vi "Cam_project_ROI.vi"() -> ()   [LabVIEW 2018]
uses:
  <vilib>/userdefined/High Color/IMAQdx.ctl
  <vilib>/vision/driver/NI_Vision_Acquisition_Software.lvlib
panel:
  out "Frame Rate 2":dbl
  out "error out":errorcluster
  out "Acquired Frames/s":dbl
  out "Distance of the object":dbl
  out "Frame Rate":dbl(knob) scale=0.0..10.0
  out "Case":cluster{i32, i32}(graph)
  out "Detection":cluster{i16, i16}(graph)
  out "cluster":T1
  out "Array":i32[](array[numeric])
  out "Numeric":i32
  out "Area of the Bounding Rectangle":i32
  out "?":T2(plugin-control)
  out "Binary Image":T2(plugin-control)
  out "?":bool
  in  "?":dbl(slide)=100.0 scale=0.0..1000.0
  out "?":T3(array[cluster]) {"Score" format="%.2f"; "Centroid"."y" format="%.2f"; "Centroid"."x" format="%.2f"}
  out "Detected:":i32
  in  "Stop":bool
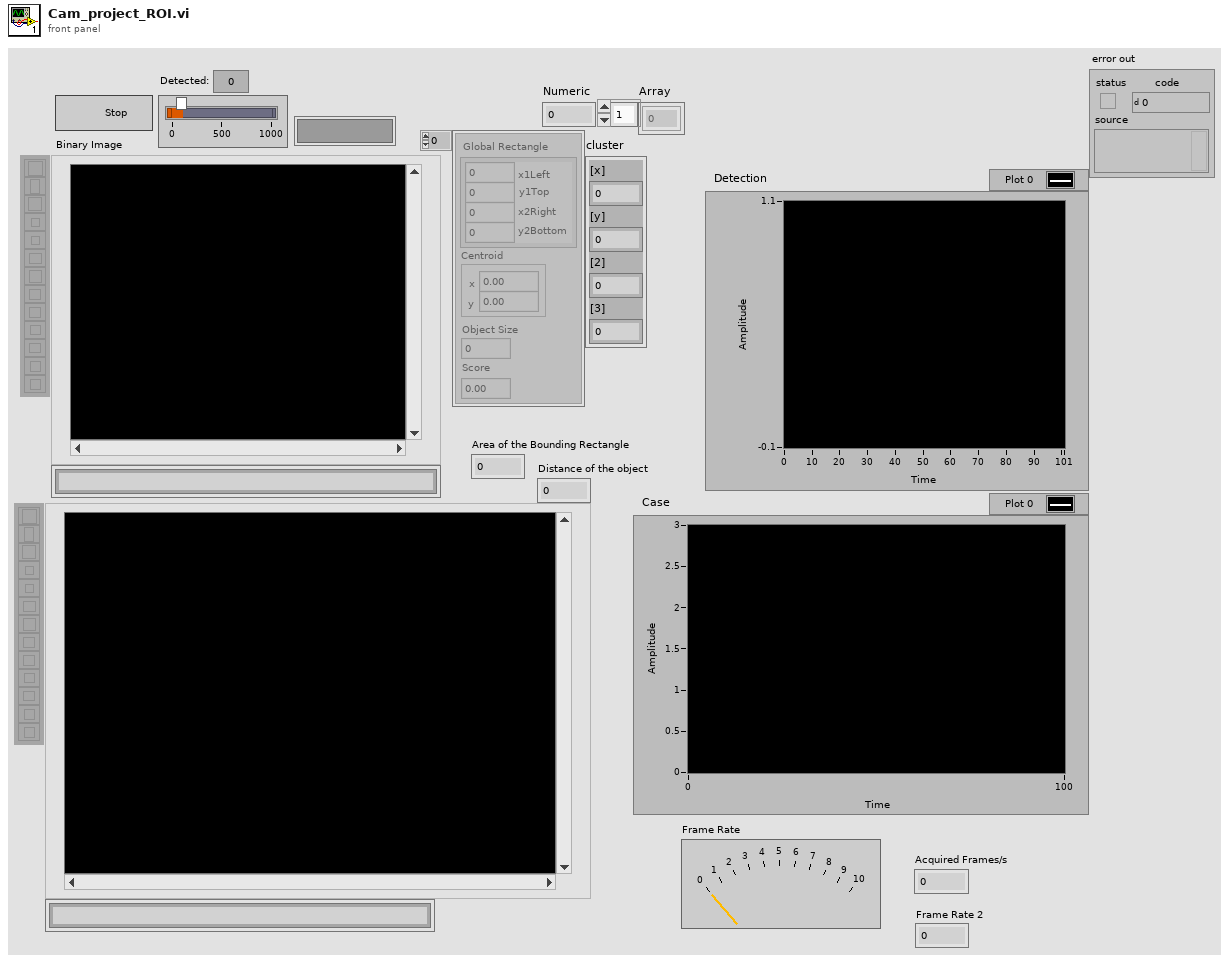
[diagram p1: front panel]
types:
  T1 = cluster{"[x]":sgl, "[y]":sgl, "[2]":sgl, "[3]":sgl}
  T2 = typedef "IMAQ Image.ctl" = refnum<image>
  T3 = cluster{"Global Rectangle":cluster{"x1Left":i32, "y1Top":i32, "x2Right":i32, "y2Bottom":i32}, "Centroid":cluster{"x":sgl, "y":sgl}, "Object Size":u32, "Score":dbl}[]
  T4 = typedef "IMAQdx.ctl" = refnum<k21>
  T5 = cluster{"Desired Font (Application)":enum16{"User-specified Font", "Application Font", "System Font", "Dialog Font"}, "[User-specified Font]":cluster{"Font Name":string, "Size":i16, "Strikeout?":bool, "Italic?":bool, "Underline?":bool, "Outline?":bool, "Shadow?":bool, "Bold?":bool, "Rotation Angle":dbl}, "Horizontal Alignment":i16, "Vertical Alignment":i16}
  T6 = enum32{"No Selection", "Point", "Line", "Rectangle", "Oval", "Polygon", "Free", "Unused1", "Unused2", "Unused3", "Broken Line", "Free Hand Line"}
  T7 = cluster{"[0]":sgl, "[1]":sgl, "[2]":sgl, "[3]":sgl}
  T8 = cluster{"[0]":dbl, "[1]":dbl, "[2]":dbl, "[3]":dbl}
  T9 = cluster{"ID":enum32{"External", "Internal"}, "Type":enum32{"No Selection", "Point", "Line", "Rectangle", "Oval", "Polygon", "Free", "Unused1", "Unused2", "Unused3", "Broken Line", "Free Hand Line"}, dbl[]}
  T10 = cluster{"ID":enum32{"External", "Internal"}, "Type":enum32{"No Selection", "Point", "Line", "Rectangle", "Oval", "Polygon", "Free", "Unused1", "Unused2", "Unused3", "Broken Line", "Free Hand Line"}, dbl[]}[]
  T11 = cluster{dbl[], cluster{"ID":enum32{"External", "Internal"}, "Type":enum32{"No Selection", "Point", "Line", "Rectangle", "Oval", "Polygon", "Free", "Unused1", "Unused2", "Unused3", "Broken Line", "Free Hand Line"}, dbl[]}[]}
  T12 = cluster{"Shape Report (Shape Detect)[0]":cluster{"Global Rectangle":cluster{"x1Left":i32, "y1Top":i32, "x2Right":i32, "y2Bottom":i32}, "Centroid":cluster{"x":sgl, "y":sgl}, "Object Size":u32, "Score":dbl}, "Shape Report (Shape Detect)[1]":cluster{"Global Rectangle":cluster{"x1Left":i32, "y1Top":i32, "x2Right":i32, "y2Bottom":i32}, "Centroid":cluster{"x":sgl, "y":sgl}, "Object Size":u32, "Score":dbl}, "Shape Report (Shape Detect)[2]":cluster{"Global Rectangle":cluster{"x1Left":i32, "y1Top":i32, "x2Right":i32, "y2Bottom":i32}, "Centroid":cluster{"x":sgl, "y":sgl}, "Object Size":u32, "Score":dbl}, "Shape Report (Shape Detect)[3]":cluster{"Global Rectangle":cluster{"x1Left":i32, "y1Top":i32, "x2Right":i32, "y2Bottom":i32}, "Centroid":cluster{"x":sgl, "y":sgl}, "Object Size":u32, "Score":dbl}, "Shape Report (Shape Detect)[4]":cluster{"Global Rectangle":cluster{"x1Left":i32, "y1Top":i32, "x2Right":i32, "y2Bottom":i32}, "Centroid":cluster{"x":sgl, "y":sgl}, "Object Size":u32, "Score":dbl}, "Shape Report (Shape Detect)[5]":cluster{"Global Rectangle":cluster{"x1Left":i32, "y1Top":i32, "x2Right":i32, "y2Bottom":i32}, "Centroid":cluster{"x":sgl, "y":sgl}, "Object Size":u32, "Score":dbl}, "Shape Report (Shape Detect)[6]":cluster{"Global Rectangle":cluster{"x1Left":i32, "y1Top":i32, "x2Right":i32, "y2Bottom":i32}, "Centroid":cluster{"x":sgl, "y":sgl}, "Object Size":u32, "Score":dbl}, "Shape Report (Shape Detect)[7]":cluster{"Global Rectangle":cluster{"x1Left":i32, "y1Top":i32, "x2Right":i32, "y2Bottom":i32}, "Centroid":cluster{"x":sgl, "y":sgl}, "Object Size":u32, "Score":dbl}, "Shape Report (Shape Detect)[8]":cluster{"Global Rectangle":cluster{"x1Left":i32, "y1Top":i32, "x2Right":i32, "y2Bottom":i32}, "Centroid":cluster{"x":sgl, "y":sgl}, "Object Size":u32, "Score":dbl}}
  T13 = cluster{"x1Left":i32, "y1Top":i32, "x2Right":i32, "y2Bottom":i32}
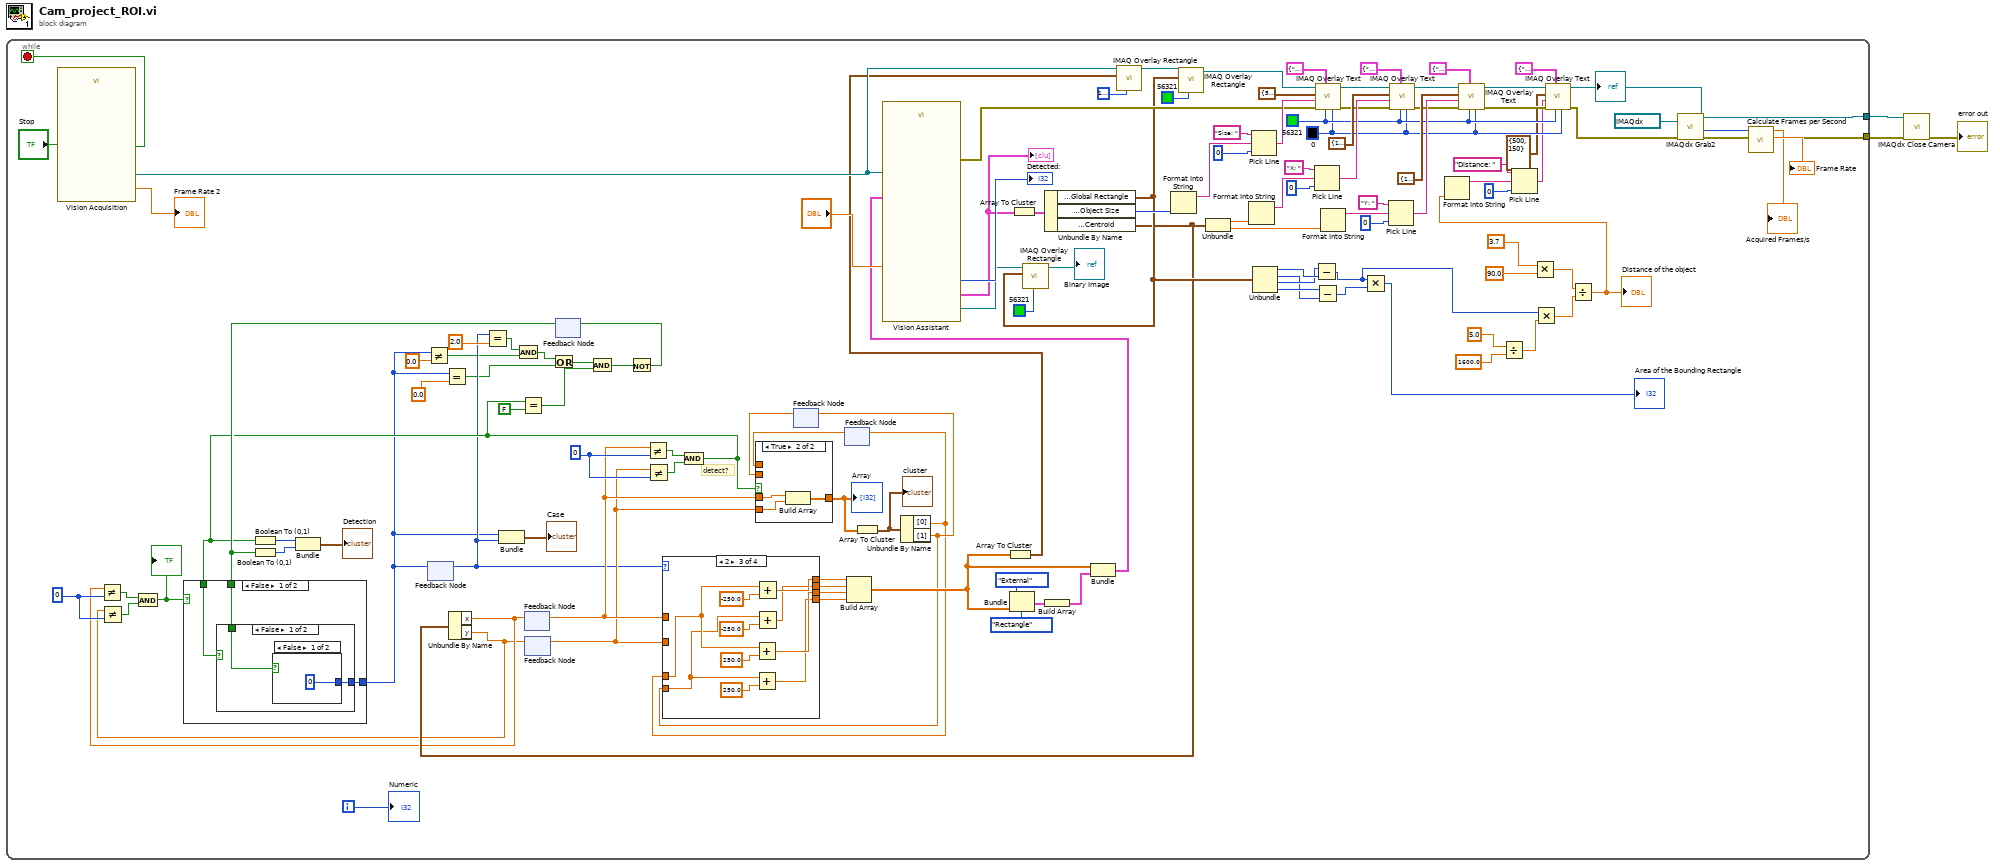
[diagram p0: block diagram]
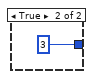
[diagram p2: hidden frame]
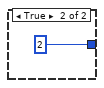
[diagram p3: hidden frame]
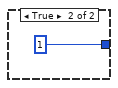
[diagram p4: hidden frame]
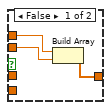
[diagram p5: hidden frame]
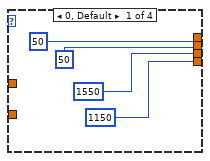
[diagram p6: hidden frame]
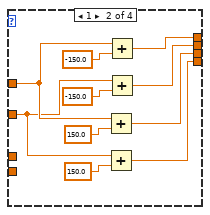
[diagram p7: hidden frame]
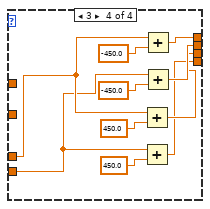
[diagram p8: hidden frame]
diagram:
  n1 = while {
    tunnel: [w8] -> w3
    tunnel: [w5] -> w2
    i -> [w56]
    stop <- w128 stop-if-true
    w66 = 0
    w71 = 0
    w17 = u32 0 ("BG Color (Transparent)")
    w18 = u32 56321 ("Text Color (black)")
    # "detect?"
    n2 = call "Vision Acquisition"("Stop (F)"="Stop") -> ("Image Out"=w81:T2, "Frame Rate"=→"Frame Rate 2":dbl, "Stopped"=w128:bool)  [unwired: 23 in, 1 out]
    n3 = feedback #1() -> (w45:i32)  [unwired: 1 in]
    n4 = Equal?(x=w45, y=sgl 2.0) -> (x = y?=w43:bool)
    n5 = feedback #2() -> (w63:sgl)  [unwired: 1 in]
    n6 = feedback #3() -> (w62:sgl)  [unwired: 1 in]
    n7 = feedback #4() -> (w52:bool)  [unwired: 1 in]
    n8 = Boolean To (0,1)(Boolean=w52) -> (0, 1=w51:i16)
    n9 = Not Equal?(x=w63, y=w66) -> (x != y?=w65:bool)
    n10 = Not Equal?(x=w62, y=w66) -> (x != y?=w64:bool)
    n11 = And(x=w65, y=w64) -> (x .and. y?=w46:bool)
    n12 = Boolean To (0,1)(Boolean=w46) -> (0, 1=w42:i16)
    n13 = Bundle(w42, w51) -> (→"Detection":cluster{i16, i16})  [unwired: 1 in]
    n14 = Equal?(x=w46, y=FALSE) -> (x = y?=w55:bool)
    n15 = feedback #5() -> (w59:sgl)  [unwired: 1 in]
    n16 = feedback #6() -> (w60:sgl)  [unwired: 1 in]
    n17 = case shown="True" w46 {
      tunnel: w63 -> [_ w143]
      tunnel: w62 -> [_ w142]
      tunnel: [w140 w141] -> w61
      tunnel: w60 -> [w138 _]
      tunnel: w59 -> [w139 _]
      frame False {
        n18 = Build Array(w138, w139) -> (w140:sgl[])
      }
      frame True {
        n19 = Build Array(w143, w142) -> (w141:sgl[])
      }
    }
    "Array" <- w61
    n20 = Array To Cluster(array=w61) -> (cluster=w33:T7)
    "cluster" <- w33
    n21 = Unbundle By Name(w33) -> ("[0]"=w57:sgl, "[1]"=w58:sgl)
    n22 = case shown="2" w45 {
      tunnel: [50 ("line index") w156 w163 w171] -> w77
      tunnel: [50 ("line index") w154 w162 w170] -> w76
      tunnel: [1550 ("line index") w150 w161 w169] -> w75
      tunnel: [1150 ("line index") w151 w160 w168] -> w74
      tunnel: w63 -> [_ w149 _ _]
      tunnel: w62 -> [_ w148 _ _]
      tunnel: w58 -> [_ _ w158 w172]
      tunnel: w57 -> [_ _ w159 w173]
      frame 0, Default {
      }
      frame 1 {
        n23 = Add(x=w149, y=150.0) -> (x+y=w150:dbl)
        n24 = Add(x=w148, y=150.0) -> (x+y=w151:dbl)
        n25 = Add(x=w149, y=-150.0) -> (x+y=w156:dbl)
        n26 = Add(x=w148, y=-150.0) -> (x+y=w154:dbl)
      }
      frame 2 {
        n27 = Add(x=w159, y=250.0) -> (x+y=w161:dbl)
        n28 = Add(x=w158, y=250.0) -> (x+y=w160:dbl)
        n29 = Add(x=w159, y=-250.0) -> (x+y=w163:dbl)
        n30 = Add(x=w158, y=-250.0) -> (x+y=w162:dbl)
      }
      frame 3 {
        n31 = Add(x=w173, y=450.0) -> (x+y=w169:dbl)
        n32 = Add(x=w172, y=450.0) -> (x+y=w168:dbl)
        n33 = Add(x=w173, y=-450.0) -> (x+y=w171:dbl)
        n34 = Add(x=w172, y=-450.0) -> (x+y=w170:dbl)
      }
    }
    n35 = feedback-in #5(w58) -> ()
    n36 = feedback-in #6(w57) -> ()
    n37 = Build Array(w77, w76, w75, w74) -> (w82:dbl[])
    n38 = Array To Cluster(array=w82) -> (cluster=w78:T8)
    n39 = Bundle("ID"=enum32{"External", "Internal"}."External", "Type"=T6."Rectangle", w82) -> (w85:T9)  [unwired: 1 in]
    n40 = Build Array(w85) -> (w84:T10)
    n41 = Bundle(w82, w84) -> (w83:T11)  [unwired: 1 in]
    n42 = call "Vision Assistant"("Image In"=w81, "Minimal Score (Shape Detect)"="?", "ROI Descriptor (Define ROI)"=w83) -> ("Image Out"=w92:T2, "Number of Matches (Shape Detect)"=→"Detected:":i32, "Shape Report (Shape Detect)"=w123:T3, "error out"=w90:errorcluster)  [unwired: 21 in]
    "?" <- w123
    n43 = Array To Cluster(array=w123) -> (cluster=w124:T12)
    n44 = Unbundle By Name(w124) -> ("Shape Report (Shape Detect)[0].Global Rectangle"=w68:T13, "Shape Report (Shape Detect)[0].Object Size"=w121:u32, "Shape Report (Shape Detect)[0].Centroid"=w67:cluster{"x":sgl, "y":sgl})
    n45 = Unbundle By Name(w67) -> ("x"=w49:sgl, "y"=w48:sgl)
    n46 = Not Equal?(x=w49, y=w71) -> (x != y?=w70:bool)
    n47 = Not Equal?(x=w48, y=w71) -> (x != y?=w69:bool)
    n48 = And(x=w70, y=w69) -> (x .and. y?=w47:bool)
    "?" <- w47
    n49 = case shown="False" w47 {
      tunnel: [w131 1] -> w39
      tunnel: w52 -> [w129 _]
      tunnel: w46 -> [w130 _]
      frame False {
        n50 = case shown="False" w130 {
          tunnel: [w133 2] -> w131
          tunnel: w129 -> [w132 _]
          frame False {
            n51 = case shown="False" w132 {
              tunnel: [0 3] -> w133
              frame False {
              }
              frame True {
              }
            }
          }
          frame True {
          }
        }
      }
      frame True {
      }
    }
    n52 = Not Equal?(x=w39, y=0.0) -> (x != y?=w38:bool)
    n53 = feedback-in #1(w39) -> ()
    n54 = Equal?(x=w39, y=0.0) -> (x = y?=w36:bool)
    n55 = Bundle(w39, w45) -> (→"Case":cluster{i32, i32})  [unwired: 1 in]
    n56 = And(x=w43, y=w38) -> (x .and. y?=w37:bool)
    n57 = feedback-in #2(w49) -> ()
    n58 = feedback-in #3(w48) -> ()
    n59 = Or(x=w37, y=w36) -> (x .or. y?=w35:bool)
    n60 = And(x=w35, y=w55) -> (x .and. y?=w41:bool)
    n61 = Not(x=w41) -> (.not. x?=w34:bool)
    n62 = feedback-in #4(w34) -> ()
    n63 = call "IMAQ Overlay Rectangle"("Color"=u32 56321, "Rectangle"=w68, "Image"=w92) -> ("Image Out"=→"Binary Image":T2)  [unwired: 7 in, 1 out]
    n64 = call "IMAQ Overlay Rectangle"("Color"=u32 16777224, "Rectangle"=w78, "Image"=w81) -> ("Image Out"=w80:T2)  [unwired: 7 in, 1 out]
    n65 = Format Into String(w121) -> (resulting string=w117:string)  [unwired: 3 in, 1 out]
    n66 = call "IMAQ Overlay Rectangle"("Color"=u32 56321, "Rectangle"=w68, "Image"=w80) -> ("Image Out"=w119:T2)  [unwired: 7 in, 1 out]
    n67 = Unbundle(w67) -> ("x"=w73:sgl, "y"=w72:sgl)
    n68 = Format Into String(w73) -> (resulting string=w105:string)  [unwired: 3 in, 1 out]
    n69 = Pick Line(string ("")="Size: ", multi-line string=w117, line index=0) -> (output string=w116:string)
    n70 = Unbundle(w68) -> ("x1Left"=w98:i32, "y1Top"=w95:i32, "x2Right"=w97:i32, "y2Bottom"=w96:i32)
    n71 = Pick Line(string ("")="X: ", multi-line string=w105, line index=0) -> (output string=w104:string)
    n72 = Subtract(x=w97, y=w98) -> (x-y=w22:i32)
    n73 = Subtract(x=w96, y=w95) -> (x-y=w99:i32)
    n74 = call "IMAQ Overlay Text"("BG Color (Transparent)"=w17, "Text Color (black)"=w18, "Font, Size & Style"=T5 {"Desired Font (Application)"=enum."System Font", "[User-specified Font]"={"Font Name"="", "Size"=15, "Strikeout?"=FALSE, "Italic?"=FALSE, "Underline?"=FALSE, "Outline?"=FALSE, "Shadow?"=FALSE, "Bold?"=TRUE, "Rotation Angle"=0.0}, "Horizontal Alignment"=0, "Vertical Alignment"=0}, "error in (no error)"=w90, "String"=w116, "Origin"=cluster{"X":i32, "Y":i32} {"X"=500, "Y"=100}, "Image"=w119) -> ("error out"=w89:errorcluster, "Image Out"=w113:T2)  [unwired: 3 in]
    n75 = Format Into String(w72) -> (resulting string=w101:string)  [unwired: 3 in, 1 out]
    n76 = Multiply(x=w22, y=w99) -> (x*y=→"Area of the Bounding Rectangle":i32)
    n77 = Pick Line(string ("")="Y: ", multi-line string=w101, line index=0) -> (output string=w102:string)
    n78 = call "IMAQ Overlay Text"("BG Color (Transparent)"=w17, "Text Color (black)"=w18, "Font, Size & Style"=T5 {"Desired Font (Application)"=enum."System Font", "[User-specified Font]"={"Font Name"="", "Size"=15, "Strikeout?"=FALSE, "Italic?"=FALSE, "Underline?"=FALSE, "Outline?"=FALSE, "Shadow?"=FALSE, "Bold?"=TRUE, "Rotation Angle"=0.0}, "Horizontal Alignment"=0, "Vertical Alignment"=0}, "error in (no error)"=w89, "String"=w104, "Origin"=cluster{"X":i32, "Y":i32} {"X"=100, "Y"=100}, "Image"=w113) -> ("error out"=w88:errorcluster, "Image Out"=w110:T2)  [unwired: 3 in]
    n79 = call "IMAQ Overlay Text"("BG Color (Transparent)"=w17, "Text Color (black)"=w18, "Font, Size & Style"=T5 {"Desired Font (Application)"=enum."System Font", "[User-specified Font]"={"Font Name"="", "Size"=15, "Strikeout?"=FALSE, "Italic?"=FALSE, "Underline?"=FALSE, "Outline?"=FALSE, "Shadow?"=FALSE, "Bold?"=TRUE, "Rotation Angle"=0.0}, "Horizontal Alignment"=0, "Vertical Alignment"=0}, "error in (no error)"=w88, "String"=w102, "Origin"=cluster{"X":i32, "Y":i32} {"X"=100, "Y"=150}, "Image"=w110) -> ("error out"=w16:errorcluster, "Image Out"=w20:T2)  [unwired: 3 in]
    n80 = Divide(x=5.0, y=1600.0) -> (x/y=w25:dbl)
    n81 = Multiply(x=3.7, y=90.0) -> (x*y=w24:dbl)
    n82 = Multiply(x=w22, y=w25) -> (x*y=w23:dbl)
    n83 = Divide(x=w24, y=w23) -> (x/y=w12:dbl)
    "Distance of the object" <- w12
    n84 = Format Into String(w12) -> (resulting string=w14:string)  [unwired: 3 in, 1 out]
    n85 = Pick Line(string ("")="Distance: ", multi-line string=w14, line index=0) -> (output string=w11:string)
    n86 = call "IMAQ Overlay Text"("BG Color (Transparent)"=w17, "Text Color (black)"=w18, "Font, Size & Style"=T5 {"Desired Font (Application)"=enum."System Font", "[User-specified Font]"={"Font Name"="", "Size"=15, "Strikeout?"=FALSE, "Italic?"=FALSE, "Underline?"=FALSE, "Outline?"=FALSE, "Shadow?"=FALSE, "Bold?"=TRUE, "Rotation Angle"=0.0}, "Horizontal Alignment"=0, "Vertical Alignment"=0}, "error in (no error)"=w16, "String"=w11, "Origin"=cluster{"X":i32, "Y":i32} {"X"=500, "Y"=150}, "Image"=w20) -> ("error out"=w6:errorcluster, "Image Out"=w19:T2)  [unwired: 3 in]
    "?" <- w19
    n87 = call <vilib>:"IMAQdx Grab2.vi"("error in"=w6, "Image In"=w19, "Session In"=T4 "cam1") -> ("error out"=w5:errorcluster, "Buffer Number Out"=w30:u32, "Session Out"=w8:T4)  [unwired: 5 in, 1 out]
    n88 = call <vilib>:"Calculate Frames per Second.vi"("Buffer Number"=w30) -> ("Processed Frames/s"=→"Frame Rate":dbl, "Acquired Frames/s"=→"Acquired Frames/s":dbl)  [unwired: 8 in, 1 out]
    "Numeric" <- w56
  }
  n89 = call <vilib>:"IMAQdx Close Camera.vi"("error in"=w2, "Session In"=w3) -> ("error out"=→"error out":errorcluster)  [unwired: 9 out]
